vi "SendFloat.vi"(5 "Sent Data":dbl, 6 "Timeout ms":i32, 7 "UDP Input":T1) -> (0 "Error Out":errorcluster, 3 "UDP Output":T1)   [LabVIEW 2019]
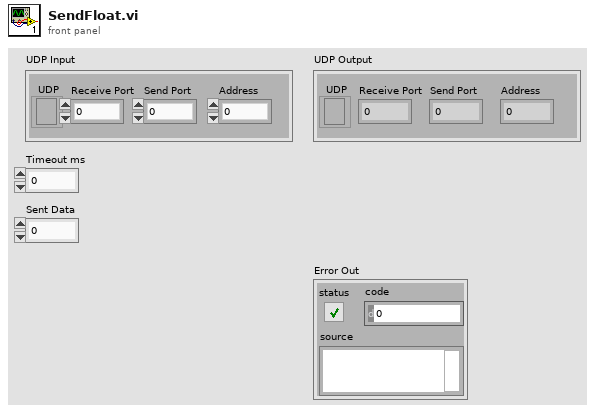
[diagram p1: front panel]
types:
  T1 = cluster{"UDP":refnum<k16>, "Receive Port":i32, "Send Port":i32, "Address":i64}
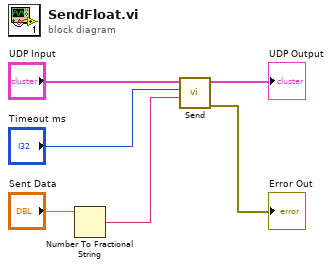
[diagram p0: block diagram]
diagram:
  n1 = Number To Fractional String(number="Sent Data") -> (F-format string=w3:string)  [unwired: 3 in]
  n2 = call "Send.vi"("SentData"=w3, "Timeout ms"="Timeout ms", "UDP Input"="UDP Input") -> ("Error Out"=→"Error Out":errorcluster, "UDP Output"=→"UDP Output":T1)  [unwired: 3 in]
